vi "Path Builder.vi"(4 "Edit? (F)":bool, 5 "Reverse Path":bool, 6 "Waypoints":cluster{dbl[], dbl[]}, 7 "Field Settings":T1={"Exchange Left"=102.0, "Exchange Right"=150.0, "Power Cube Zone Left"=139.5, "Power Cube Zone Right"=139.5, "Switch Left"=85.25, "Switch Right"=85.25, "Switch Front"=140.0, "Switch Back"=196.0, "Platform Left"=95.25, "Platform Right"=95.25, "Platform Front"=261.47, "Slalom Depth"=235.235}, 8 "Robot width (in)":dbl=34.0, 9 "y start":dbl, 10 "Start Point":cluster{"x":dbl, "y":dbl}, 11 "Field":cluster{dbl[], dbl[]}[](array[cluster])) -> (0 "Reverse Path?":bool, 1 "Waypoints":cluster{dbl[], dbl[]}, 2 "Graph Path":cluster{dbl[], dbl[]}, 3 "Path":cluster{"x":dbl, "y":dbl}[](array[cluster]))   [LabVIEW 2018]
uses:
  Typedef/Field Settings.ctl
panel:
  in  "Points":cluster{"X":dbl, "Y":dbl}[](array[cluster])
  out "Field Half":cluster{dbl[], dbl[]}[](graph)
  in  "Done":bool
  in  "Cancel":bool
  in  "Clear":bool
  in  "Generate":bool
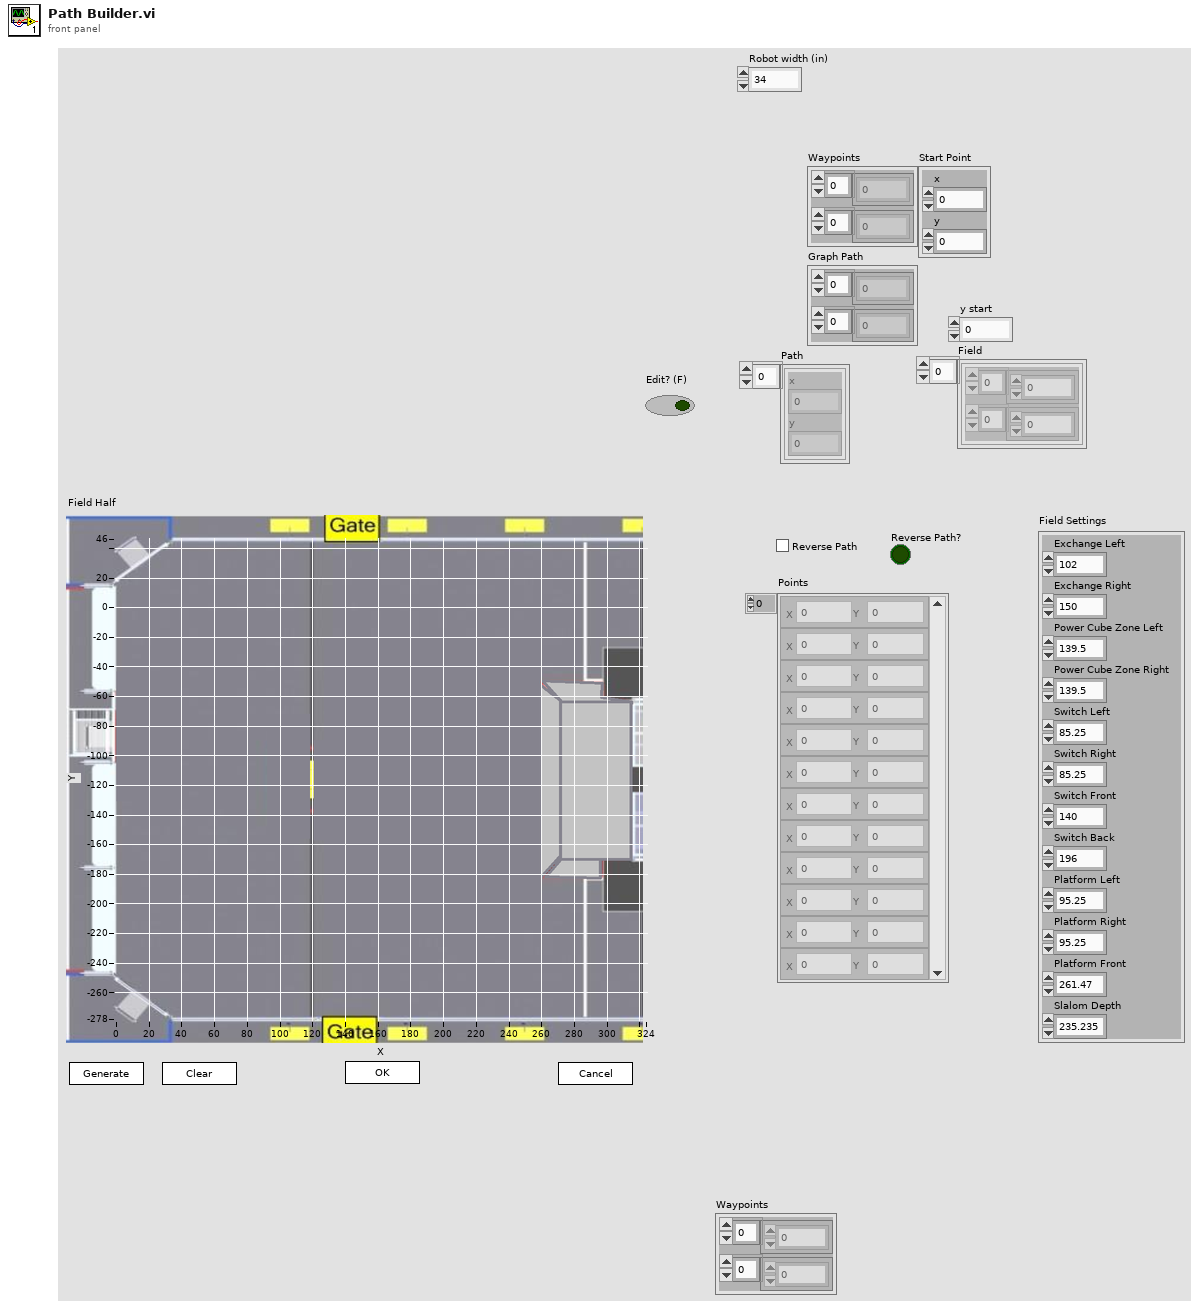
[diagram p1: front panel]
types:
  T1 = typedef "Field Settings.ctl" = cluster{"Exchange Left":dbl, "Exchange Right":dbl, "Power Cube Zone Left":dbl, "Power Cube Zone Right":dbl, "Switch Left":dbl, "Switch Right":dbl, "Switch Front":dbl, "Switch Back":dbl, "Platform Left":dbl, "Platform Right":dbl, "Platform Front":dbl, "Slalom Depth":dbl}
  T2 = typedef "LVPoint32TypeDef.ctl" = cluster{"Horizontal":i32, "Vertical":i32}
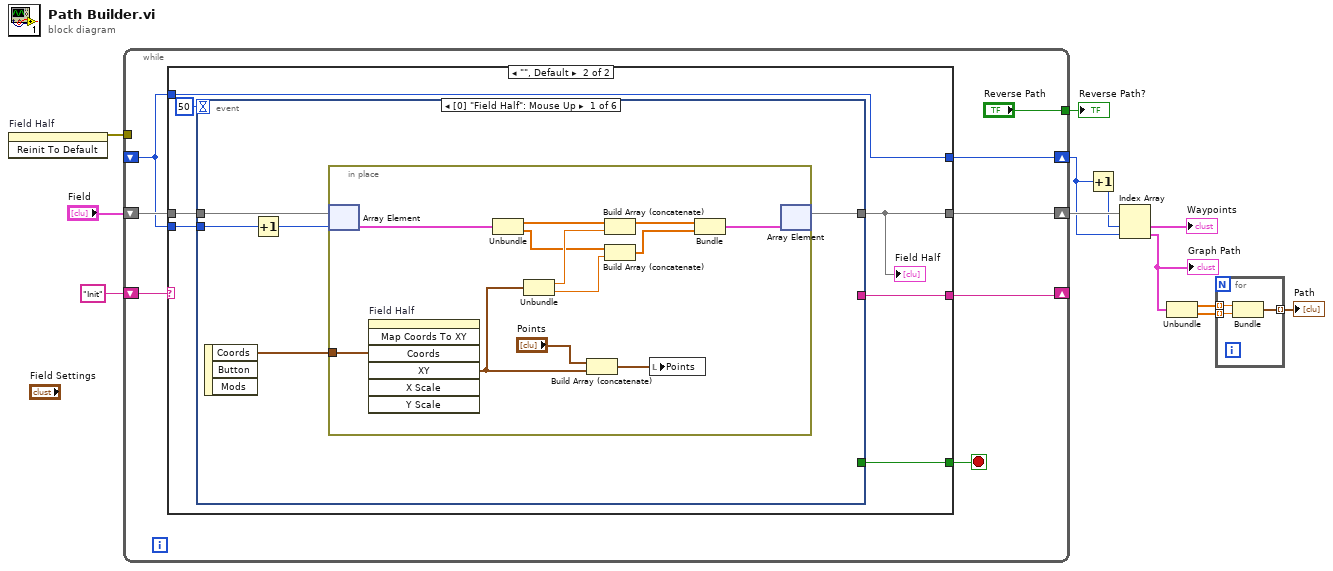
[diagram p0: block diagram]
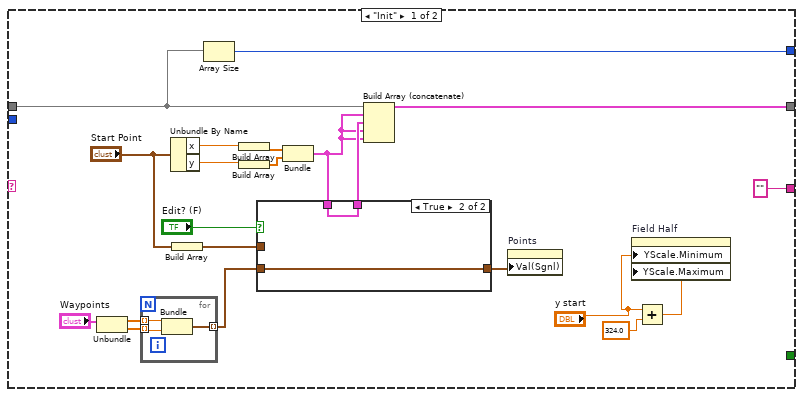
[diagram p2: hidden frame]
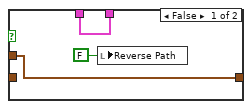
[diagram p3: hidden frame]
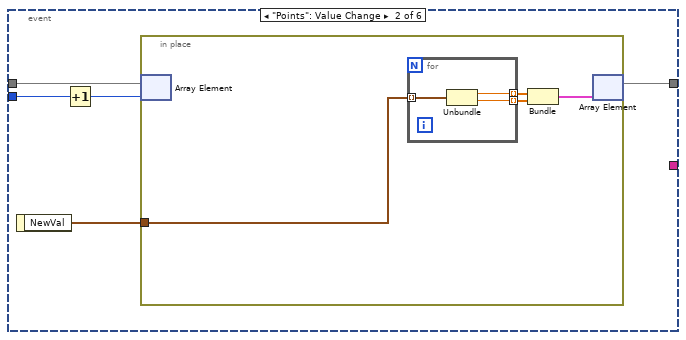
[diagram p4: hidden frame]
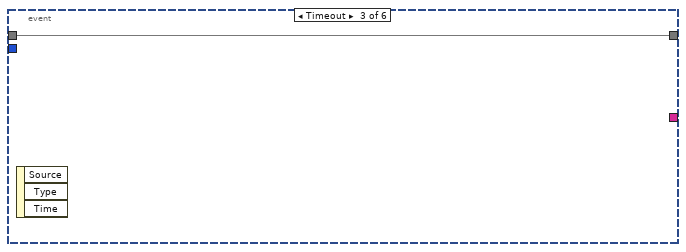
[diagram p5: hidden frame]
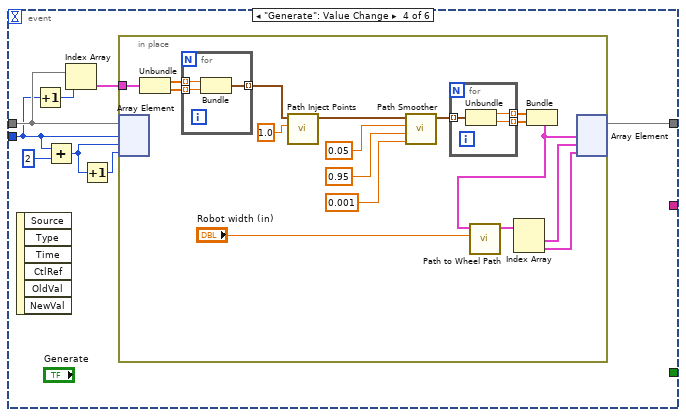
[diagram p6: hidden frame]
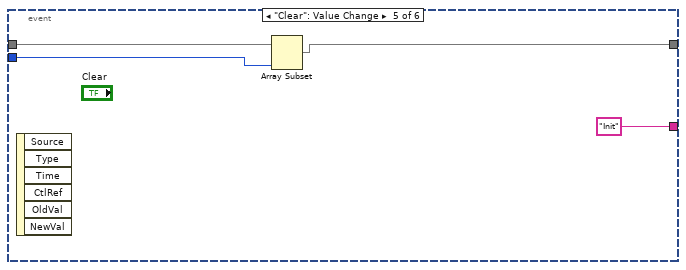
[diagram p7: hidden frame]
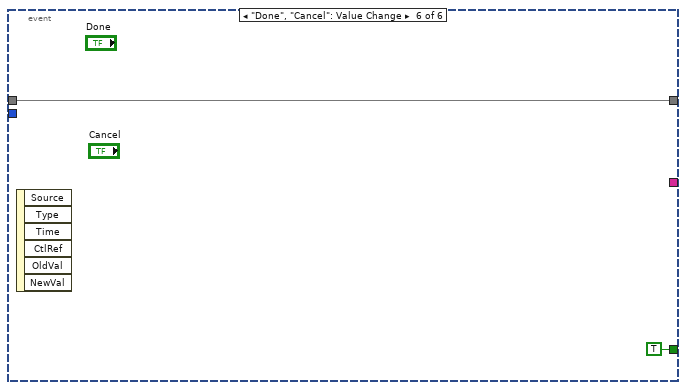
[diagram p8: hidden frame]
diagram:
  n1 = invoke on="Field Half" class="XYGraph (strict)" method="Reinit To Default"() -> (error out=w8:errorcluster)  [unwired: 3 in, 2 out]
  n2 = while {
    shift-right: [w19] -> w11
    shift-left: "Field" -> [w20]
    shift-right: [w17] -> _
    shift-left: "Init" -> [w18]
    tunnel: w8 -> [_]
    shift-right: [w15] -> w7
    shift-left: _ -> [w14]
    tunnel: ["Reverse Path"] -> w1
    stop <- w16 stop-if-true
    n3 = case shown="\"\", Default" w18 {
      tunnel: w20 -> [w35 w56]
      tunnel: [w36 w51] -> w19
      tunnel: ["" w55] -> w17
      tunnel: [_ w54] -> w16
      tunnel: [w34 w53] -> w15
      tunnel: w14 -> [_ w53]
      tunnel: w14 -> [_ w52]
      frame "Init" {
        n4 = Unbundle("Waypoints") -> (w23:dbl[], w22:dbl[])
        n5 = for {
          tunnel: w23 -> [w44] mode=indexing
          tunnel: w22 -> [w43] mode=indexing
          tunnel: [w42] -> w21 mode=indexing
          n6 = Bundle("x"=w44, "y"=w43) -> (w42:cluster{"x":dbl, "y":dbl})  [unwired: 1 in]
        }
        n7 = Unbundle By Name("Start Point") -> ("x"=w40:dbl, "y"=w39:dbl)
        n8 = Build Array("Start Point") -> (w26:cluster{"x":dbl, "y":dbl}[])
        n9 = Array Size(array=w35) -> (size(s)=w34:i32)
        n10 = Build Array(w40) -> (w38:dbl[])
        n11 = Build Array(w39) -> (w37:dbl[])
        n12 = Bundle(w38, w37) -> (w27:cluster{dbl[], dbl[]})  [unwired: 1 in]
        n13 = case shown="True" "Edit? (F)" {
          tunnel: [w47 w49] -> w28
          tunnel: w27 -> [w47 w49]
          tunnel: w21 -> [_ w48]
          tunnel: [w46 w48] -> w25
          tunnel: w26 -> [w46 _]
          frame False {
            n14 = local write "Reverse Path"(FALSE ("Reverse Path")) -> ()
          }
          frame True {
          }
        }
        n15 = Build Array (concatenate)(w35, w27, w28, w27, w27) -> (w36:cluster{dbl[], dbl[]}[])
        n16 = property on="Points" class="Arr (strict)"("Val(Sgnl)"=w25) -> ()  [unwired: 2 in, 2 out]
        n17 = Add(x="y start", y=324.0 ("x")) -> (x+y=w32:dbl)
        n18 = property on="Field Half" class="XYGraph (strict)"("YScale.Minimum"="y start", "YScale.Maximum"=w32) -> ()  [unwired: 2 in, 2 out]
      }
      frame "", Default {
        n19 = event shown="[0] \"Field Half\": Mouse Up" {
          selector: _ -> [_ _ _ _ _ _]
          dyn-events: _ -> [_ _ _ _ _ _]
          timeout: 50 -> [_ _ _ _ _ _]
          tunnel: w56 -> [w61 w78 w86 w93 w119 w122]
          tunnel: [w59 w77 w86 w94 w118 w122] -> w51
          tunnel: [_ _ _ _ "Init" _] -> w55
          tunnel: [_ _ _ _ _ TRUE] -> w54
          tunnel: w52 -> [w58 w76 _ w89 w120 _]
          event "Field Half": Mouse Up {
            n20 = event-data() -> ("Coords"=w60:T2)  [unwired: 1 in, 2 out]
            n21 = Increment(x=w58) -> (x+1=w57:i32)
            n22 = in-place {
              in-place-border: w60 -> [w65]
              n23 = in-place-array #1(w61, w57) -> (w73:cluster{dbl[], dbl[]})
              n24 = invoke on="Field Half" class="XYGraph (strict)" method="Map Coords To XY"("Coords"=w65) -> ("XY"=w63:cluster{"X":dbl, "Y":dbl})  [unwired: 6 in, 6 out]
              n25 = Unbundle(w73) -> (w71:dbl[], w70:dbl[])
              n26 = Unbundle(w63) -> ("X"=w72:dbl, "Y"=w69:dbl)
              n27 = Build Array (concatenate)("Points", w63) -> (w62:cluster{"X":dbl, "Y":dbl}[])
              n28 = Build Array (concatenate)(w71, w72) -> (w68:dbl[])
              n29 = Build Array (concatenate)(w70, w69) -> (w67:dbl[])
              n30 = local write "Points"(w62) -> ()
              n31 = Bundle(w68, w67) -> (w66:cluster{dbl[], dbl[]})  [unwired: 1 in]
              n32 = in-place-array #1(w66) -> (w59:cluster{dbl[], dbl[]}[])  [unwired: 1 out]
            }
          }
          event "Points": Value Change {
            n33 = event-data() -> ("NewVal"=w74:cluster{"X":dbl, "Y":dbl}[])  [unwired: 1 in]
            n34 = Increment(x=w76) -> (x+1=w75:i32)
            n35 = in-place {
              in-place-border: w74 -> [w82]
              n36 = in-place-array #2(w78, w75) -> ()  [unwired: 1 out]
              n37 = for {
                tunnel: w82 -> [w85] mode=indexing
                tunnel: [w84] -> w81 mode=indexing
                tunnel: [w83] -> w80 mode=indexing
                n38 = Unbundle(w85) -> ("X"=w84:dbl, "Y"=w83:dbl)
              }
              n39 = Bundle(w81, w80) -> (w79:cluster{dbl[], dbl[]})  [unwired: 1 in]
              n40 = in-place-array #2(w79) -> (w77:cluster{dbl[], dbl[]}[])  [unwired: 1 out]
            }
          }
          event Timeout {
            n41 = event-data() -> ()  [unwired: 1 in, 3 out]
          }
          event "Generate": Value Change {
            n42 = event-data() -> ()  [unwired: 1 in, 6 out]
            n43 = Increment(x=w89) -> (x+1=w91:i32)
            n44 = Add(x=w89, y=2) -> (x+y=w88:i32)
            n45 = Index Array(array=w93, index=w91) -> (element=w92:cluster{dbl[], dbl[]})
            n46 = Increment(x=w88) -> (x+1=w90:i32)
            n47 = in-place {
              in-place-border: w92 -> [w111]
              n48 = in-place-array #3(w93, w89, w88, w90) -> ()  [unwired: 3 out]
              n49 = Unbundle(w111) -> (w110:dbl[], w109:dbl[])
              n50 = for {
                tunnel: w110 -> [w117] mode=indexing
                tunnel: w109 -> [w116] mode=indexing
                tunnel: [w115] -> w103 mode=indexing
                n51 = Bundle("x"=w117, "y"=w116) -> (w115:cluster{"x":dbl, "y":dbl})  [unwired: 1 in]
              }
              n52 = call "Path Inject Points.vi"("Distance"=1.0, "Path"=w103) -> ("Path out"=w108:cluster{dbl, dbl}[])  [unwired: 9 in]
              n53 = call "Path Smoother.vi"("tolerance"=0.001, "B"=0.95, "A"=0.05, "Path"=w108) -> ("SmoothPath"=w102:cluster{dbl, dbl}[])  [unwired: 7 in]
              n54 = for {
                tunnel: w102 -> [w114] mode=indexing
                tunnel: [w113] -> w100 mode=indexing
                tunnel: [w112] -> w101 mode=indexing
                n55 = Unbundle(w114) -> (w113:dbl, w112:dbl)
              }
              n56 = Bundle(w100, w101) -> (w98:cluster{dbl[], dbl[]})  [unwired: 1 in]
              n57 = call "Path to Wheel Path.vi"("Wheelbase (in)"="Robot width (in)", "waypoints"=w98) -> ("out"=w97:cluster{dbl[], dbl[]}[])  [unwired: 9 in]
              n58 = Index Array(array=w97) -> (element #1=w96:cluster{dbl[], dbl[]}, element #2=w95:cluster{dbl[], dbl[]})  [unwired: 2 in]
              n59 = in-place-array #3(w98, w96, w95) -> (w94:cluster{dbl[], dbl[]}[])  [unwired: 3 out]
            }
          }
          event "Clear": Value Change {
            n60 = event-data() -> ()  [unwired: 1 in, 6 out]
            n61 = Array Subset(array=w119, length=w120) -> (w118:cluster{dbl[], dbl[]}[])  [unwired: 1 in]
          }
          event "Done", "Cancel": Value Change {
            n62 = event-data() -> ()  [unwired: 1 in, 6 out]
          }
        }
        "Field Half" <- w51
      }
    }
  }
  "Reverse Path?" <- w1
  n63 = Increment(x=w7) -> (x+1=w6:i32)
  n64 = Index Array(array=w11, index #1=w6, index #2=w7) -> (element #1=→"Waypoints":cluster{dbl[], dbl[]}, element #2=w5:cluster{dbl[], dbl[]})
  "Graph Path" <- w5
  n65 = Unbundle(w5) -> (w4:dbl[], w3:dbl[])
  n66 = for {
    tunnel: w4 -> [w126] mode=indexing
    tunnel: w3 -> [w125] mode=indexing
    tunnel: [w124] -> w2 mode=indexing
    n67 = Bundle("x"=w126, "y"=w125) -> (w124:cluster{"x":dbl, "y":dbl})  [unwired: 1 in]
  }
  "Path" <- w2
